vi "Dynamixel Multi Function.vi"(6 "Data Array":u32[](array[numeric]), 7 "Function Array":T1[](array[typedef]), 8 "Model Number":u32, 10 "Motor ID":u8[](array[numeric]), 11 "Com port":refnum<visa-resource-name> caption="instrument handle") -> (0 "error out":errorcluster, 2 "Function Return":i32[](array[numeric]))   [LabVIEW 2022 SP3]
uses:
  Sub Vis/Dynamixel Commands.ctl
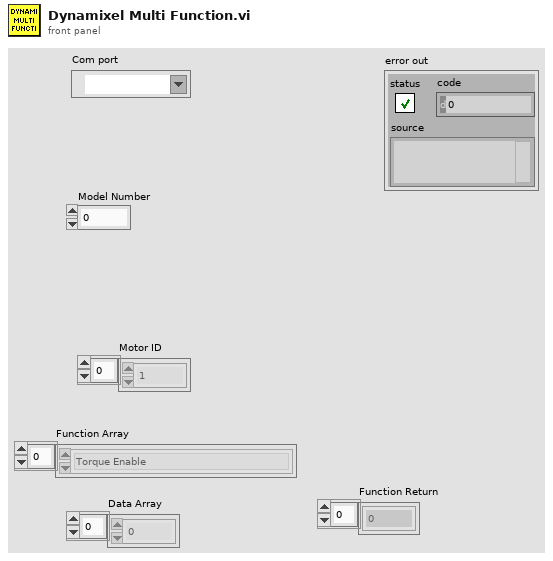
[diagram p1: front panel]
types:
  T1 = typedef "Dynamixel Commands.ctl" = enum16{"Torque Enable", "Present Position", "Threshold", "Max Position Limit", "Acceleration Profile", "Velocity Profile", "Goal Position", "Position Proportional Gain", "Position Integral Gain", "Position Differential Gain ", "Shutdown", "Write Operating Mode", "Read Operating Mode"}
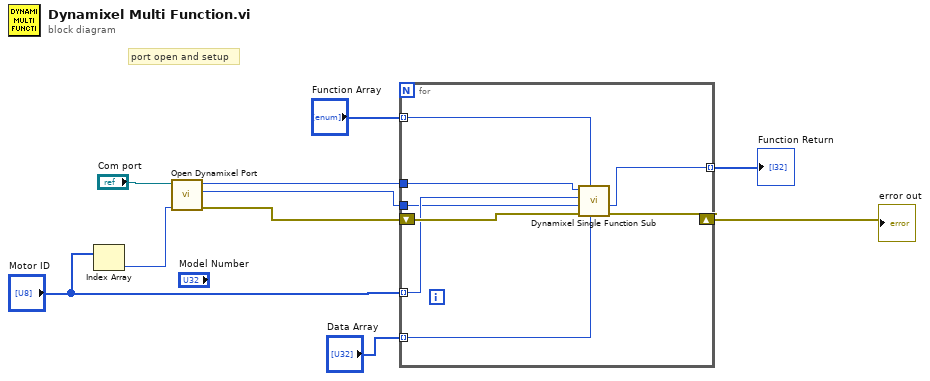
[diagram p0: block diagram]
diagram:
  # "port open and setup"
  n1 = Index Array(array="Motor ID") -> (element=w2:u8)  [unwired: 1 in]
  n2 = call "Open Dynamixel Port.vi"("dynamixel_id"=w2, "Com port"="Com port") -> ("error out"=w6:errorcluster, "Model Number"=w1:u32, "port_num"=w5:i32)  [unwired: 7 in]
  n3 = for {
    shift-right: [w17] -> w4
    shift-left: w6 -> [w18]
    tunnel: "Function Array" -> [w15] mode=indexing
    tunnel: "Data Array" -> [w14] mode=indexing
    tunnel: "Motor ID" -> [w16] mode=indexing
    tunnel: [w13] -> w8 mode=indexing
    tunnel: w5 -> [w12]
    tunnel: w1 -> [w11]
    n4 = call "Dynamixel Single Function Sub.vi"("data"=w14, "Function"=w15, "error In"=w18, "Model Number"=w11, "dynamixel_id"=w16, "port_num"=w12) -> ("error out"=w17:errorcluster, "Value returned"=w13:i32)  [unwired: 4 in]
  }
  "error out" <- w4
  "Function Return" <- w8
